vi "Set AQ Parameters.vi"(8 "error in":errorcluster, 9 "Señal Digital":T1={"Puertos/Pines"="", "Puerto"="DAQSim1", "Pines"=[], "Tiempo de AQ"=0.0, "Tiempo entre AQ"=0.0}, 10 "Señal Analogica":T2={"Canal"="DAQSim1", "Canales"=[], "Frecuencia de muestreo"=1000, "Numero de muestras"=1000, "Tiempo de AQ"=0.0, "Canal/Canales"=""}) -> (0 "error out":errorcluster)   [LabVIEW 2020, in "Aqcisition.lvlib"]
doc: "It will indicate what are we going to see\n_____\nCreated using Delacor QMH Event Scripter 6.0.0.121."
uses:
  Aqcisition.lvlib
  Analog Signal Config.ctl
  Digital Signal Config.ctl
  Set AQ Parameters Argument--cluster.ctl
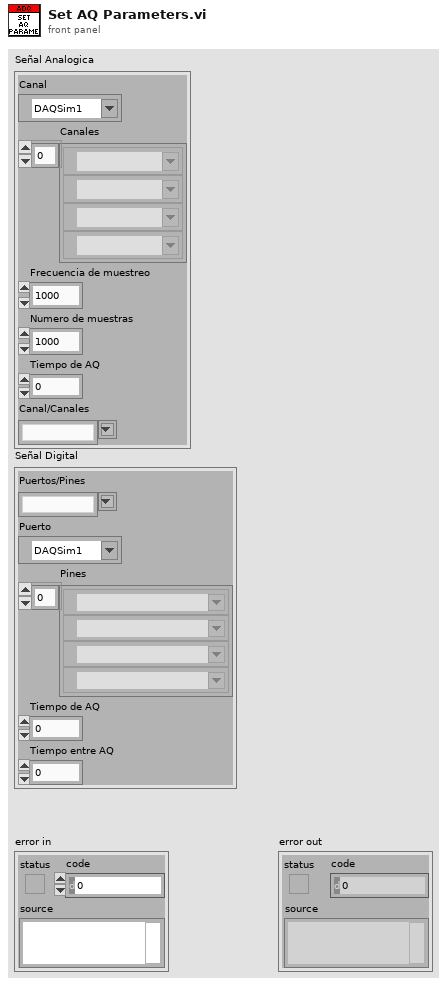
[diagram p1: front panel]
types:
  T1 = typedef "Digital Signal Config.ctl" = cluster{"Puertos/Pines":string, "Puerto":tag, "Pines":tag[], "Tiempo de AQ":dbl, "Tiempo entre AQ":dbl}
  T2 = typedef "Analog Signal Config.ctl" = cluster{"Canal":tag, "Canales":tag[], "Frecuencia de muestreo":i32, "Numero de muestras":i32, "Tiempo de AQ":dbl, "Canal/Canales":string}
  T3 = typedef "Aqcisition.lvlib/Set AQ Parameters Argument--cluster.ctl" = cluster{"Señal Analogica":T2, "Señal Digital":T1}
  T4 = typedef "Aqcisition.lvlib/Request Events--cluster.ctl" = cluster{"Stop Module":refnum<user-event>, "Show Panel":refnum<user-event>, "Hide Panel":refnum<user-event>, "Get Module Execution Status":refnum<user-event>, "Show Diagram":refnum<user-event>, "Start Adqcisition":refnum<user-event>, "Stop Adqcisition":refnum<user-event>, "Wake Up Helper Loop":refnum<user-event>, "Put HL to Sleep":refnum<user-event>, "Set AQ Parameters":refnum<user-event>, "Wake up Digital Loop":refnum<user-event>}
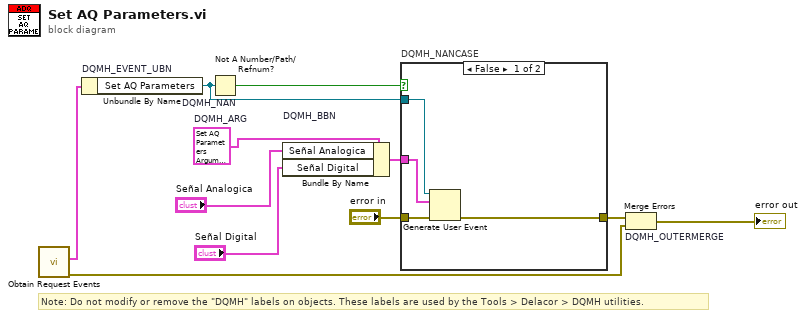
[diagram p0: block diagram]
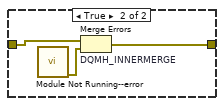
[diagram p2: hidden frame]
diagram:
  w5 = T3 {"Señal Analogica"={"Canal"="DAQSim1", "Canales"=[], "Frecuencia de muestreo"=1000, "Numero de muestras"=1000, "Tiempo de AQ"=0.0, "Canal/Canales"=""}, "Señal Digital"={"Puertos/Pines"="", "Puerto"="DAQSim1", "Pines"=[], "Tiempo de AQ"=0.0, "Tiempo entre AQ"=0.0}}  # DQMH_ARG
  # "Note: Do not modify or remove the \"DQMH\" labels on objects. These labels are used by the Tools > Delacor > DQMH utilities."
  n1 = call "Obtain Request Events.vi"() -> ("error out"=w2:errorcluster, "Aqcisition Request Events"=w1:T4)  [unwired: 10 in]
  n2 = Unbundle By Name "DQMH_EVENT_UBN"(w1) -> ("Set AQ Parameters"=w7:refnum<user-event>)
  n3 = Not A Number/Path/Refnum? "DQMH_NAN"(number/path/refnum=w7) -> (NaN/Path/Refnum?=w8:bool)
  n4 = Bundle By Name "DQMH_BBN"(cluster=w5, "Señal Analogica"="Señal Analogica", "Señal Digital"="Señal Digital") -> (w9:T3)
  n5 = case "DQMH_NANCASE" shown="False" w8 {
    tunnel: "error in" -> [w15 w18]
    tunnel: [w14 w17] -> w6
    tunnel: w7 -> [w13 _]
    tunnel: w9 -> [w12 _]
    frame False {
      n6 = Generate User Event(user event=w13, event data cluster=w12, error in=w15) -> (error out=w14:errorcluster)  [unwired: 1 in, 1 out]
    }
    frame True {
      n7 = call "Module Not Running--error.vi"() -> ("error out"=w16:errorcluster)  [unwired: 11 in]
      n8 = Merge Errors "DQMH_INNERMERGE"(w18, w16) -> (w17:errorcluster)
    }
  }
  n9 = Merge Errors "DQMH_OUTERMERGE"(w6, w2) -> (→"error out":errorcluster)
